vi "opencvFindPeakTest.vi"   [LabVIEW 2017]
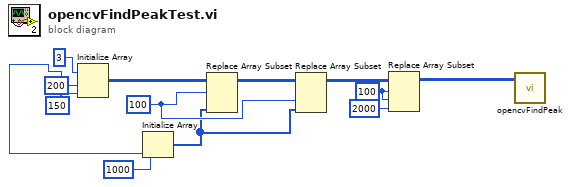
[diagram p0: block diagram]
diagram:
  w3 = 100 ("index (row)")
  w8 = 100 ("index (row)")
  w6 = 150 ("dimension size")
  n1 = Initialize Array(u16 3 ("element"), 200 ("dimension size"), w6) -> (w11:u16[][])
  n2 = Initialize Array(u16 1000 ("element"), w6) -> (w7:u16[])
  n3 = Replace Array Subset(array=w11, new element=w7, index (row)=w8) -> (w9:u16[][])  [unwired: 1 in]
  n4 = Replace Array Subset(array=w9, new element=w7, index (col)=w8) -> (w4:u16[][])  [unwired: 1 in]
  n5 = Replace Array Subset(array=w4, new element=u16 2000 ("new element/subarray"), index (row)=w3, index (col)=w3) -> (w1:u16[][])
  n6 = call "opencvFindPeak.vi"("Image (2D)"=w1) -> ()  [unwired: 1 in, 2 out]
